vi "SailSuggestionsUpperLevelTest.vi"() -> ()   [LabVIEW 2012]
panel:
  out "Did any VIs raise flags?":bool[](array[boolean])
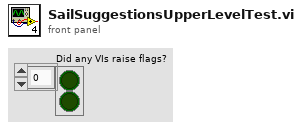
[diagram p1: front panel]
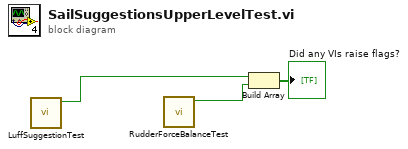
[diagram p0: block diagram]
diagram:
  n1 = call "LuffSuggestionTest.vi"() -> ("Were there any errors at all?"=w2:bool)  [unwired: 11 in]
  n2 = call "RudderForceBalanceTest.vi"() -> ("Were there any errors at all?"=w3:bool)  [unwired: 11 in]
  n3 = Build Array(w2, w3) -> (→"Did any VIs raise flags?":bool[])
